vi "Errror on bit.vi"(8 "error in (no error)":errorcluster, 11 "RFID system in":refnum<class "RFID system.lvclass">) -> (0 "error out":errorcluster, 2 "Error on  byte":dbl, 3 "RFID system out":refnum<class "RFID system.lvclass">)   [LabVIEW 2019, in "RFID system.lvclass"]
uses:
  RFID system.lvclass
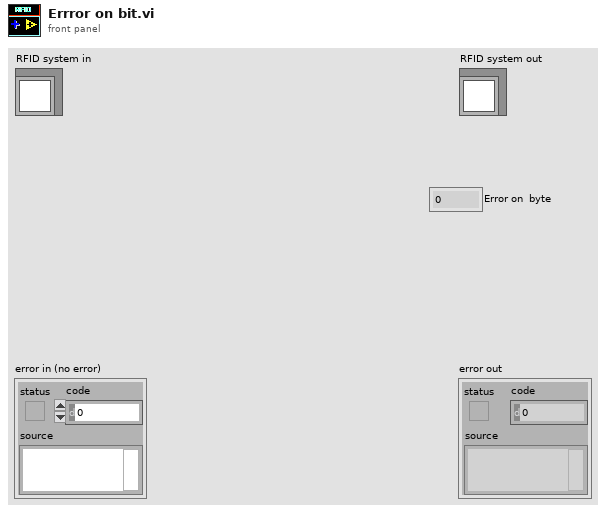
[diagram p1: front panel]
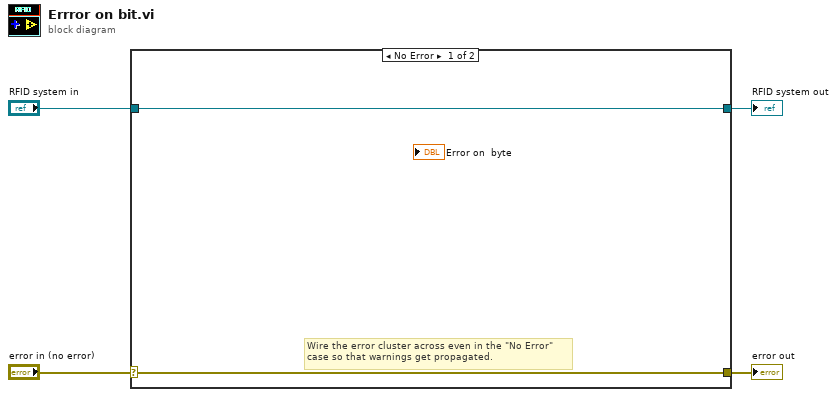
[diagram p0: block diagram]
diagram:
  n1 = case shown="No Error" "error in (no error)" {
    selector: "error in (no error)" -> [w6 w8]
    tunnel: [w6 w8] -> w3
    tunnel: [w5 w7] -> w1
    tunnel: "RFID system in" -> [w5 w7]
    frame No Error {
      # "Wire the error cluster across even in the \"No Error\"\ncase so that warnings get propagated."
    }
    frame Error {
    }
  }
  "error out" <- w3
  "RFID system out" <- w1
